vi "Get or Add NumberingFormats.vi"(8 "error in":errorcluster, 11 "SpreadsheetDoc in":refnum<k24>) -> (0 "error out":errorcluster, 2 "NumberingFormats":refnum<k24>, 3 "SpreadsheetDoc out":refnum<k24>)   [LabVIEW 2021, in "Open Xml.lvlib"]
uses:
  Open Xml.lvlib
  D:/git/Open-Xml-LabVIEW/dll/DocumentFormat.OpenXml.dll
  dll/DocumentFormat.OpenXml.dll
  D:/git/Open-Xml-LabVIEW/dll/DocumentFormat.OpenXml.Framework.dll
  dll/DocumentFormat.OpenXml.Framework.dll
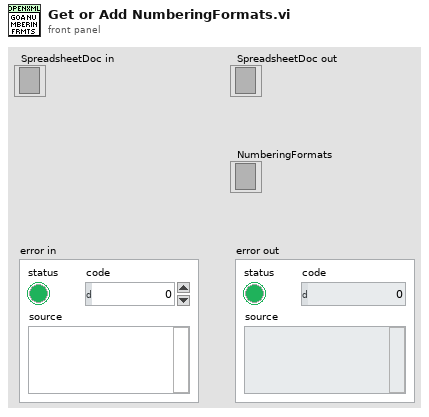
[diagram p1: front panel]
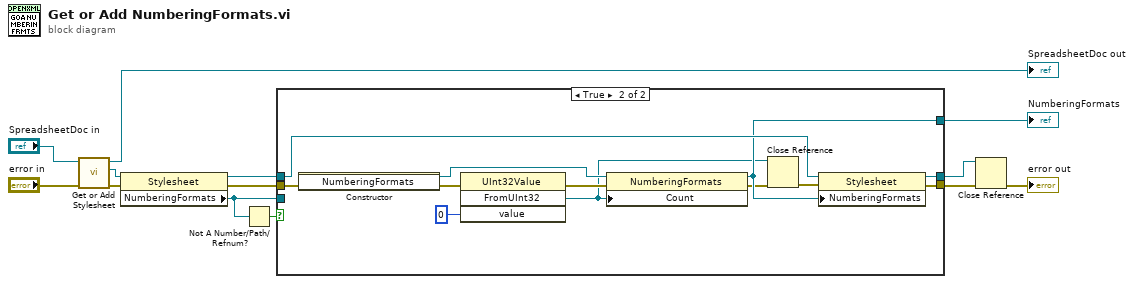
[diagram p0: block diagram]
diagram:
  n1 = call "Get or Add Stylesheet.vi"("error in"="error in", "SpreadsheetDoc in"="SpreadsheetDoc in") -> ("error out"=w4:errorcluster, "Stylesheet"=w6:refnum<k24>, "SpreadsheetDoc out"=→"SpreadsheetDoc out":refnum<k24>)  [unwired: 7 in]
  n2 = property class="Stylesheet"(reference=w6, error in=w4) -> (reference out=w11:refnum<k24>, error out=w8:errorcluster, "NumberingFormats"=w10:refnum<k24>)
  n3 = Not A Number/Path/Refnum?(number/path/refnum=w10) -> (NaN/Path/Refnum?=w7:bool)
  n4 = case shown="True" w7 {
    tunnel: w8 -> [w14 w28]
    tunnel: w10 -> [w15 _]
    tunnel: w11 -> [w16 w27]
    tunnel: [w14 w25] -> w12
    tunnel: [w16 w26] -> w2
    tunnel: [w15 w22] -> w1
    frame False {
    }
    frame True {
      n5 = constructor class="NumberingFormats"(error in=w28) -> (reference out=w24:refnum<k24>, error out=w21:errorcluster)  [unwired: 2 in, 1 out]
      n6 = invoke class="UInt32Value" method="FromUInt32"(error in=w21, "value"=u32 0) -> (error out=w20:errorcluster, "FromUInt32"=w19:refnum<k24>)  [unwired: 2 in, 2 out]
      n7 = property class="NumberingFormats"(reference=w24, error in=w20, "Count"=w19) -> (reference out=w22:refnum<k24>, error out=w18:errorcluster)
      n8 = Close Reference(reference=w19, error in (no error)=w18) -> (error out=w17:errorcluster)
      n9 = property class="Stylesheet"(reference=w27, error in=w17, "NumberingFormats"=w22) -> (reference out=w26:refnum<k24>, error out=w25:errorcluster)
    }
  }
  "NumberingFormats" <- w1
  n10 = Close Reference(reference=w2, error in (no error)=w12) -> (error out=→"error out":errorcluster)
